vi "Tacking Helper - Data Breakdown.vi"(6 "Absolute\nWind Vector":T2, 9 "Second\nWaypoint\nPosition":T1, 10 "Boat\nPosition":T1, 11 "Waypoint\nPosition":T1) -> (1 "Angle of Wind":dbl, 2 "X, boat > wp":dbl, 3 "Y, boat >wp":dbl, 4 "Boat <> 2nd wp Angle":dbl, 5 "Boat <> wp Angle":dbl)   [LabVIEW 2011]
doc: "This vi is purely to conserve space - it is not particularly modular. It simply does the work unbundling the data and translating the (x, y) components of GPS data into usable angles."
uses:
  2 Typedefs/Velocity.ctl
  2 Typedefs/UTM Location.ctl
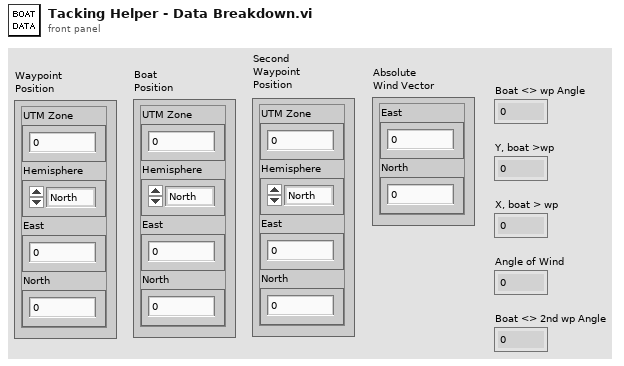
[diagram p1: front panel]
types:
  T1 = typedef "UTM Location.ctl" = cluster{"UTM Zone":dbl, "Hemisphere":enum16{"North", "South"}, "East":dbl, "North":dbl}
  T2 = typedef "Velocity.ctl" = cluster{"East":dbl, "North":dbl}
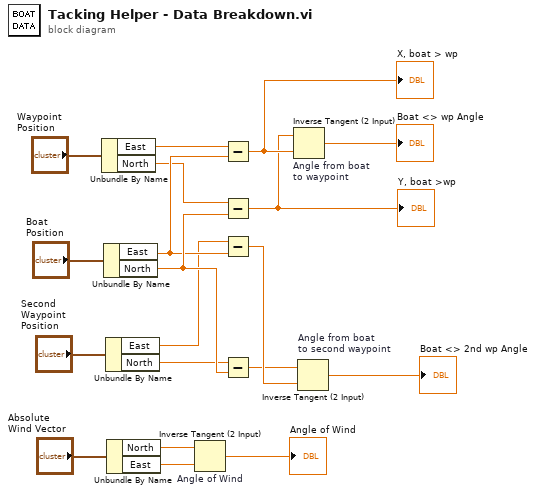
[diagram p0: block diagram]
diagram:
  n1 = Unbundle By Name("Waypoint\nPosition") -> ("East"=w1:dbl, "North"=w2:dbl)
  n2 = Unbundle By Name("Boat\nPosition") -> ("East"=w7:dbl, "North"=w9:dbl)
  n3 = Unbundle By Name("Second\nWaypoint\nPosition") -> ("East"=w6:dbl, "North"=w8:dbl)
  n4 = Unbundle By Name("Absolute\nWind Vector") -> ("North"=w3:dbl, "East"=w4:dbl)
  n5 = Inverse Tangent (2 Input) "Angle of Wind"(1:w4, 2:w3) -> (0:→"Angle of Wind":dbl)
  n6 = Subtract(x=w1, y=w7) -> (x-y=w14:dbl)
  "X, boat > wp" <- w14
  n7 = Subtract(x=w2, y=w9) -> (x-y=w13:dbl)
  "Y, boat >wp" <- w13
  n8 = Subtract(x=w6, y=w7) -> (x-y=w11:dbl)
  n9 = Subtract(x=w8, y=w9) -> (x-y=w10:dbl)
  n10 = Inverse Tangent (2 Input) "Angle from boat\nto waypoint"(1:w14, 2:w13) -> (0:→"Boat <> wp Angle":dbl)
  n11 = Inverse Tangent (2 Input) "Angle from boat\nto second waypoint"(1:w11, 2:w10) -> (0:→"Boat <> 2nd wp Angle":dbl)
